vi "Get Glyph Metrics.vi"(8 "error in (no error)":errorcluster, 11 "glyph ref in":i64) -> (0 "error out":errorcluster, 2 "metrics":T1, 3 "glyph ref out":i64)   [LabVIEW 2023, in "Freetype Drawer.lvlib"]
uses:
  Freetype Drawer.lvlib
  FT Metrics.ctl
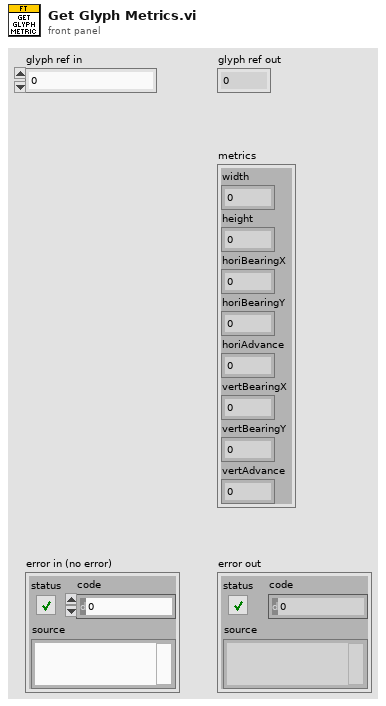
[diagram p1: front panel]
types:
  T1 = typedef "Freetype Drawer.lvlib/FT Metrics.ctl" = cluster{"width":sgl, "height":sgl, "horiBearingX":sgl, "horiBearingY":sgl, "horiAdvance":sgl, "vertBearingX":sgl, "vertBearingY":sgl, "vertAdvance":sgl}
  T2 = typedef "Freetype Drawer.lvlib/Glyph Rec.ctl" = cluster{"Library":i64, "Face":i64, "Next Glyph":i64, "glyph index":u32, "generic":cluster{"pointer":i64, "finalizer":i64}, "metrics":T3, "linearHoriAdvance":i32, "linearVertAdvance":i32, "advance":cluster{"x":i32, "y":i32}, "format":i32, "bitmap":T4, "bitmap_left":i32, "bitmap_top":i32}
  T3 = typedef "Freetype Drawer.lvlib/FT Metrics RAW.ctl" = cluster{"width":i32, "height":i32, "horiBearingX":i32, "horiBearingY":i32, "horiAdvance":i32, "vertBearingX":i32, "vertBearingY":i32, "vertAdvance":i32}
  T4 = typedef "Freetype Drawer.lvlib/FT Bitmap.ctl" = cluster{"rows":u32, "width":u32, "pitch":i32, "buffer ref":i64, "num grays":i16, "pixel_mode":u8, "palette mode":u8, "palette":i64}
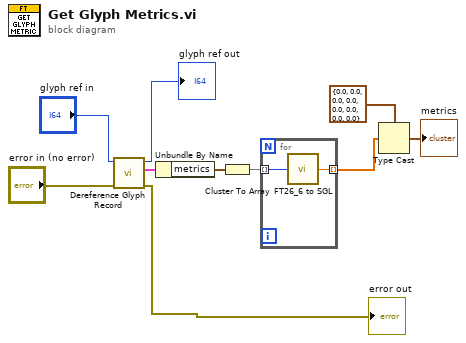
[diagram p0: block diagram]
diagram:
  n1 = call "Dereference Glyph Record.vi"("error in (no error)"="error in (no error)", "glyph ref in"="glyph ref in") -> ("error out"=→"error out":errorcluster, "out"=w8:T2, "glyph ref out"=→"glyph ref out":i64)  [unwired: 7 in]
  n2 = Unbundle By Name(w8) -> ("metrics"=w7:T3)
  n3 = Cluster To Array(cluster=w7) -> (array=w6:i32[])
  n4 = for {
    tunnel: w6 -> [w12] mode=indexing
    tunnel: [w11] -> w4 mode=indexing
    n5 = call "FT26_6 to SGL.vi"("26.6"=w12) -> ("sgl"=w11:sgl)
  }
  n6 = Type Cast(type=T1 {"width"=0.0, "height"=0.0, "horiBearingX"=0.0, "horiBearingY"=0.0, "horiAdvance"=0.0, "vertBearingX"=0.0, "vertBearingY"=0.0, "vertAdvance"=0.0} ("metrics"), x=w4) -> (*(type *) &x=→"metrics":T1)
